vi "I16.vi"(4 "Value":i16) -> (1 "Constant":refnum<class "Abs_I16 Integer.lvclass">)   [LabVIEW 2021, in "Const_I16.lvclass"]
uses:
  Const_I16.lvclass
  Abs_Types/I16 Integer/Abs_I16 Integer.lvclass
  C:/Program Files (x86)/National Instruments/LabVIEW 2021/vi.lib/TSA/Abstract Data Classes/Abs_Types/I16 Integer/Abs_I16 Integer.lvclass
  Const_I16.lvclass/Const_I16.ctl
  Properties/Write Value.vi
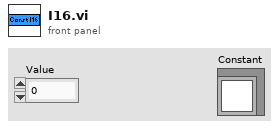
[diagram p1: front panel]
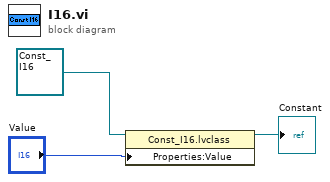
[diagram p0: block diagram]
diagram:
  n1 = property class="Const_I16.lvclass"(reference=refnum<class "Const_I16.lvclass"> refnum ("Constants.lvlib:Numeric.lvclass"), "Properties:Value"="Value") -> (reference out=→"Constant":refnum<class "Const_I16.lvclass">)  [unwired: 1 in, 1 out]
